vi "ep_1-Phase SVAF.vi"(0 "signal":dbl[](array[numeric]), 1 "reset? (F)":bool, 2 "difference? (T)":bool=TRUE, 5 "filter information":cluster{"coefficients":dbl[], "delay":i32}, 11 "error in (no error)":errorcluster, 12 "previous SVAF state":T1) -> (4 "SVAF signal":dbl[](array[numeric]), 14 "next SVAF state":T1, 15 "error out":errorcluster)   [LabVIEW 2014, in "NI_EP_Motor Monitoring.lvlib"]
uses:
  <vilib>/addons/Electrical Power/Motor Monitoring/NI_EP_Motor Monitoring.lvlib
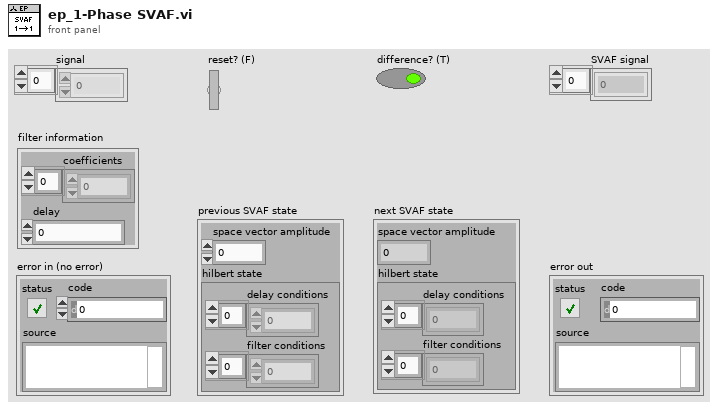
[diagram p1: front panel]
types:
  T1 = cluster{"space vector amplitude":dbl, "hilbert state":cluster{"delay conditions":dbl[], "filter conditions":dbl[]}}
  T2 = cluster{"delay conditions":dbl[], "filter conditions":dbl[]}
  T3 = cluster{"filter conditions":dbl[], "delay conditions":dbl[]}
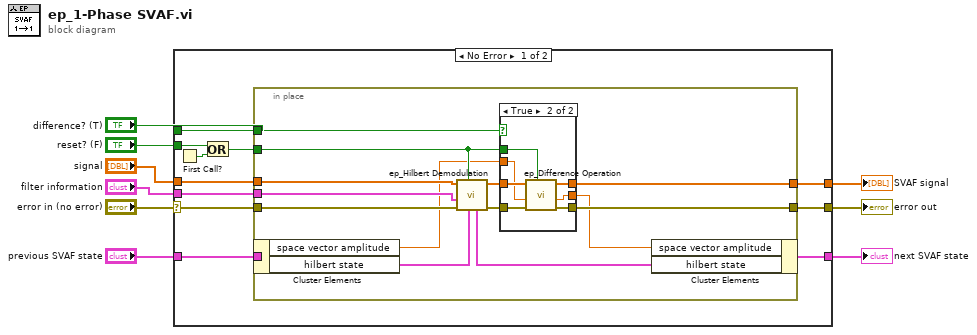
[diagram p0: block diagram]
diagram:
  n1 = case shown="No Error" "error in (no error)" {
    selector: "error in (no error)" -> [w19 w44]
    tunnel: [w12 w44] -> w3
    tunnel: "filter information" -> [w20 _]
    tunnel: "previous SVAF state" -> [w11 w43]
    tunnel: "reset? (F)" -> [w17 _]
    tunnel: [w16 _] -> w6
    tunnel: "difference? (T)" -> [w15 _]
    tunnel: [w10 w43] -> w4
    tunnel: "signal" -> [w14 _]
    frame No Error {
      n2 = First Call?() -> (First Call?: T/F=w18:bool)
      n3 = Or(x=w17, y=w18) -> (x .or. y?=w13:bool)
      n4 = in-place {
        in-place-border: w20 -> [w33]
        in-place-border: w19 -> [w32]
        in-place-border: w11 -> [_]
        in-place-border: [w30] -> w16
        in-place-border: w15 -> [w29]
        in-place-border: w14 -> [w28]
        in-place-border: w13 -> [w27]
        in-place-border: [w25] -> w12
        n5 = in-place-cluster #1(w11) -> ("space vector amplitude"=w24:dbl, "hilbert state"=w23:T2)
        n6 = call <vilib>:"ep_Hilbert Demodulation.vi"("previous state"=w23, "reset? (F)"=w27, "error in (no error)"=w32, "filter information"=w33, "signal"=w28) -> ("error out"=w26:errorcluster, "demodulated signal"=w31:dbl[], "next state"=w21:T3)  [unwired: 4 in]
        n7 = case shown="True" w29 {
          tunnel: [_ w39] -> w22
          tunnel: w24 -> [_ w41]
          tunnel: w31 -> [w35 w42]
          tunnel: [w35 w40] -> w30
          tunnel: w27 -> [_ w38]
          tunnel: w26 -> [w34 w37]
          tunnel: [w34 w36] -> w25
          frame False {
          }
          frame True {
            n8 = call <vilib>:"ep_Difference Operation.vi"("reset? (F)"=w38, "error in (no error)"=w37, "previous value"=w41, "signal in"=w42) -> ("error out"=w36:errorcluster, "next  value"=w39:dbl, "signal out"=w40:dbl[])  [unwired: 5 in]
          }
        }
        n9 = in-place-cluster #1("space vector amplitude"=w22, "hilbert state"=w21) -> (w10:T1)
      }
    }
    frame Error {
    }
  }
  "error out" <- w3
  "SVAF signal" <- w6
  "next SVAF state" <- w4
